vi "Abort Single Point Source-Ganging.vi"(8 "error in":errorcluster, 11 "Ganged Session In":T1) -> (0 "error out":errorcluster)   [LabVIEW 2021]
doc: "Abort the single point. In case of error resets the device for ganging configuration."
uses:
  controls/Abort Single Point-Ganging.ctl
  channel ganging/shared subVIs/ctl/NIDCPower_channel_ganging - ctl - ganged config.ctl
  channel ganging/shared subVIs/ctl/NIDCPower_channel_ganging - ctl - channel mode.ctl
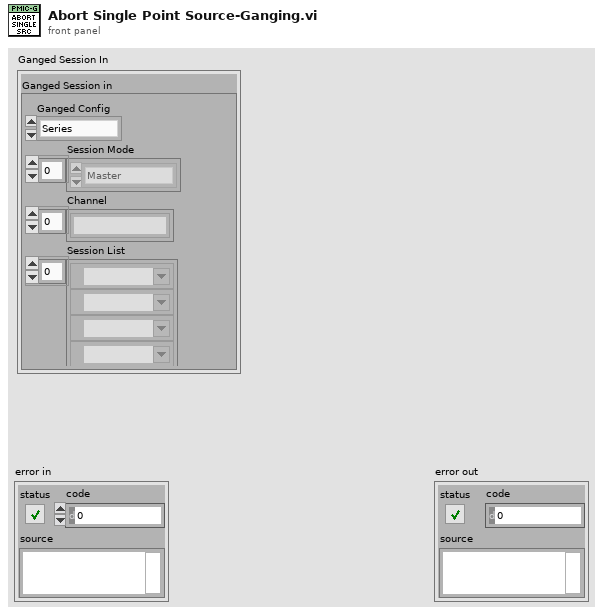
[diagram p1: front panel]
types:
  T1 = typedef "Abort Single Point-Ganging.ctl" = cluster{"Ganged Session in":cluster{"Ganged Config":T2, "Session List":refnum<k15>[], "Session Mode":T3[], "Channel":string[]}}
  T2 = typedef "NIDCPower_channel_ganging - ctl - ganged config.ctl" = enum32{"Series", "Parallel", "Manual"}
  T3 = typedef "NIDCPower_channel_ganging - ctl - channel mode.ctl" = enum32{"Master", "Slave", "Slave - Inverted"}
  T4 = cluster{"Ganged Config":T2, "Session List":refnum<k15>[], "Session Mode":T3[], "Channel":string[]}
  T5 = typedef "NIDCPower_channel_ganging - ctl - ganged session.ctl" = cluster{"Ganged Config":T2, "Session List":refnum<k15>[], "Session Mode":T3[], "Channel":string[]}
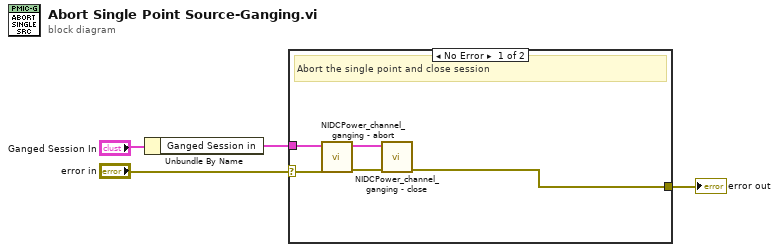
[diagram p0: block diagram]
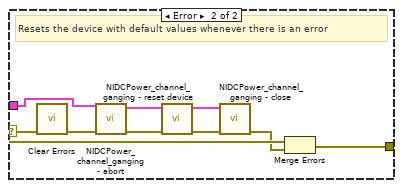
[diagram p2: hidden frame]
diagram:
  n1 = Unbundle By Name("Ganged Session In") -> ("Ganged Session in"=w1:T4)
  n2 = case shown="No Error" "error in" {
    selector: "error in" -> [w9 w12]
    tunnel: w1 -> [w5 w14]
    tunnel: [w8 w10] -> w3
    frame No Error {
      # "Abort the single point and close session"
      n3 = call "NIDCPower_channel_ganging - abort.vi"("error in (no error)"=w9, "Ganged Session In"=w5) -> ("error out"=w6:errorcluster, "Ganged Session Out"=w7:T5)  [unwired: 8 in]
      n4 = call "NIDCPower_channel_ganging - close.vi"("error in (no error)"=w6, "Ganged Session In"=w7) -> ("error out"=w8:errorcluster)  [unwired: 9 in]
    }
    frame Error {
      # "Resets the device with default values whenever there is an error"
      n5 = call <vilib>:"Clear Errors.vi"("error in (no error)"=w12) -> ("error out"=w13:errorcluster)  [unwired: 5 in, 1 out]
      n6 = call "NIDCPower_channel_ganging - abort.vi"("error in (no error)"=w13, "Ganged Session In"=w14) -> ("error out"=w17:errorcluster, "Ganged Session Out"=w18:T5)  [unwired: 8 in]
      n7 = call "NIDCPower_channel_ganging - reset device.vi"("error in (no error)"=w17, "Ganged Session In"=w18) -> ("error out"=w15:errorcluster, "Ganged Session Out"=w16:T5)  [unwired: 8 in]
      n8 = call "NIDCPower_channel_ganging - close.vi"("error in (no error)"=w15, "Ganged Session In"=w16) -> ("error out"=w11:errorcluster)  [unwired: 9 in]
      n9 = Merge Errors(w12, w11) -> (w10:errorcluster)
    }
  }
  "error out" <- w3
